vi "Construct_Optimal_Subtrack_(101-111)-1.vi"(6 "[IN] Indexes for Jumps":i32[](array[numeric]), 8 "error IN":errorcluster, 9 "[IN] Index of recon\nstructed tracks":i32, 10 "[IN] Clusters for Re\nconstructed Tracks":T1, 11 "[IN] Still connected\ntracks in group":T2) -> (0 "error OUT":errorcluster, 2 "[OUT] Clusters for Re\nconstructed Tracks":T1)   [LabVIEW 2013]
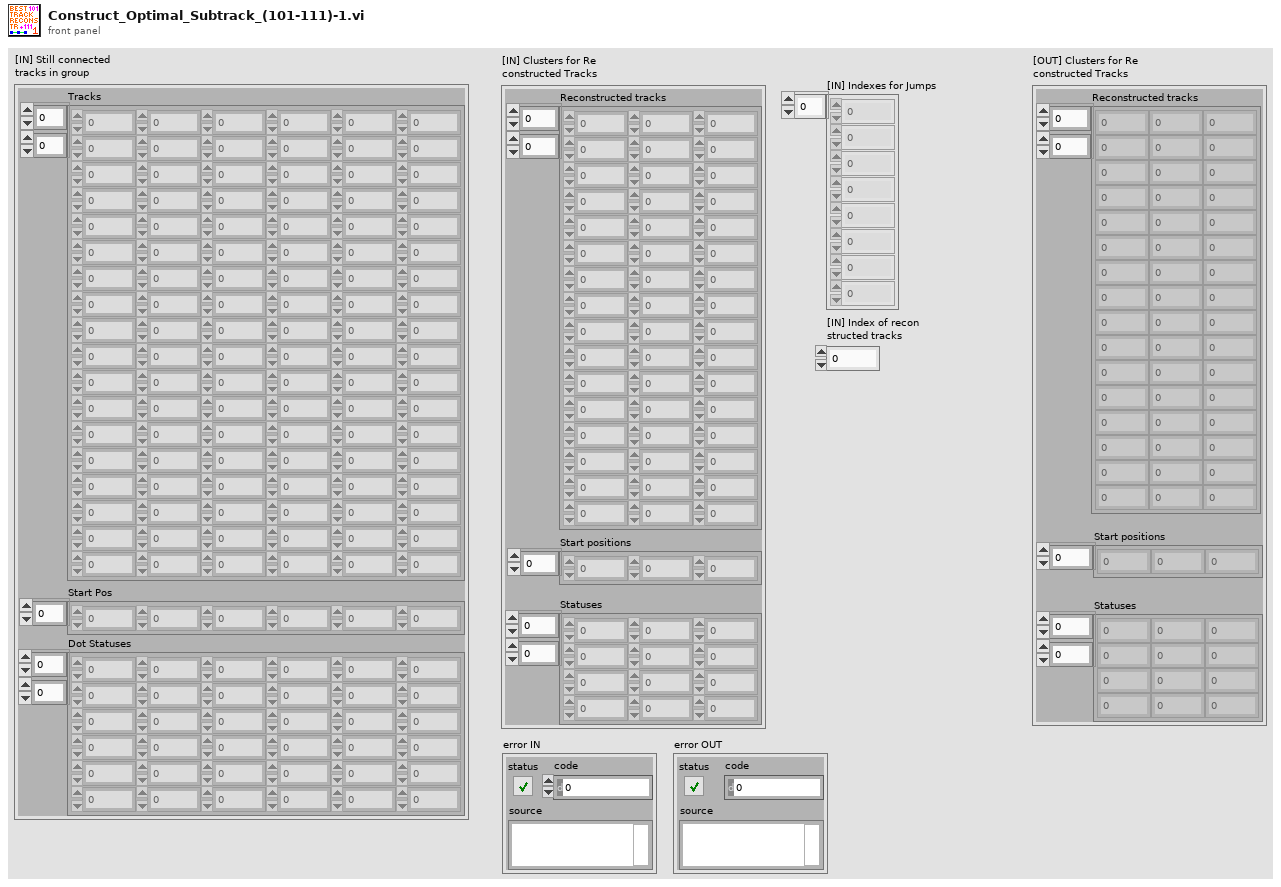
[diagram p1: front panel]
types:
  T1 = cluster{"Reconstructed tracks":dbl[][], "Start positions":i32[], "Statuses":i16[][]}
  T2 = cluster{"Tracks":dbl[][], "Start Pos":i32[], "Dot Statuses":i16[][]}
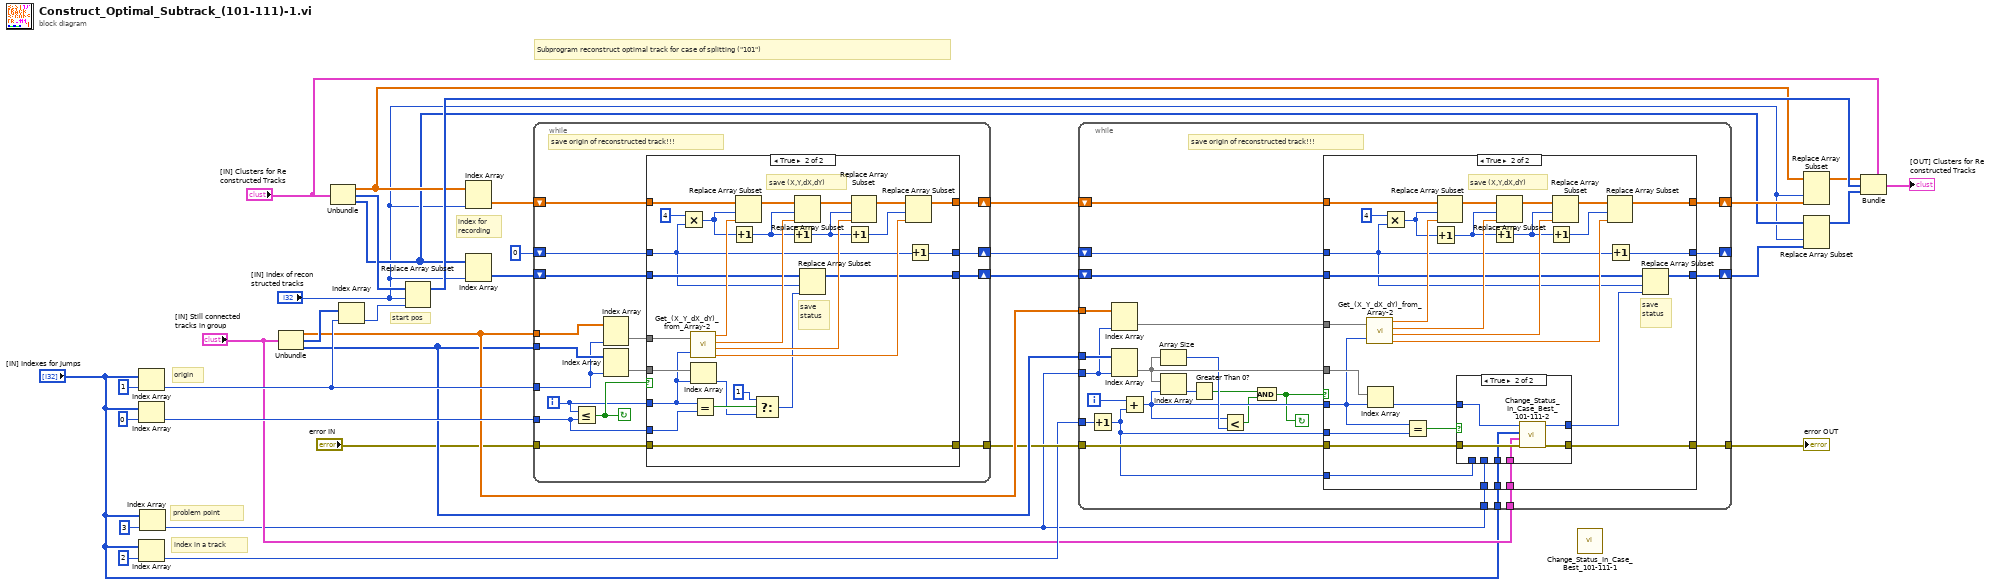
[diagram p0: block diagram]
diagram:
  # "index in a track"
  # "problem point"
  # "origin"
  # "Subprogram reconstruct optimal track for case of splitting (\"101\")"
  # "index for\nrecording"
  # "start pos"
  n1 = Index Array(array="[IN] Indexes for Jumps", index=1) -> (element=w27:i32)
  n2 = Index Array(array="[IN] Indexes for Jumps", index=0) -> (element=w30:i32)
  n3 = Index Array(array="[IN] Indexes for Jumps", index=2) -> (element=w7:i32)
  n4 = Index Array(array="[IN] Indexes for Jumps", index=3) -> (element=w3:i32)
  n5 = Unbundle("[IN] Still connected\ntracks in group") -> ("Tracks"=w19:dbl[][], "Start Pos"=w28:i32[], "Dot Statuses"=w18:i16[][])
  n6 = Unbundle("[IN] Clusters for Re\nconstructed Tracks") -> ("Reconstructed tracks"=w15:dbl[][], "Start positions"=w29:i32[], "Statuses"=w12:i16[][])
  n7 = Index Array(array=w28, index=w27) -> (element=w26:i32)
  n8 = Replace Array Subset(array=w29, new element=w26, index="[IN] Index of recon\nstructed tracks") -> (w16:i32[])
  n9 = Index Array(array=w15, index (col)="[IN] Index of recon\nstructed tracks") -> (element=w25:dbl[])  [unwired: 1 in]
  n10 = Index Array(array=w12, index (col)="[IN] Index of recon\nstructed tracks") -> (element=w24:i16[])  [unwired: 1 in]
  n11 = while {
    tunnel: w30 -> [w35]
    tunnel: w19 -> [w50]
    tunnel: w18 -> [w49]
    tunnel: w27 -> [w48]
    shift-right: [w40] -> w22
    shift-left: w25 -> [w46]
    shift-right: [w38] -> w20
    shift-left: w24 -> [w42]
    shift-right: [w39] -> w21
    shift-left: 0 -> [w41]
    tunnel: "error IN" -> [w37]
    tunnel: [w36] -> w8
    i -> [w43]
    stop <- w47 continue-if-true
    # "save origin of reconstructed track!!!"
    n12 = Less Or Equal?(x=w43, y=w35) -> (x <= y?=w47:bool)
    n13 = Index Array(array=w50, index (col)=w48) -> (element=w45:dbl[])  [unwired: 1 in]
    n14 = Index Array(array=w49, index (col)=w48) -> (element=w44:i16[])  [unwired: 1 in]
    n15 = case shown="True" w47 {
      tunnel: w46 -> [w54 w79]
      tunnel: w45 -> [_ w81]
      tunnel: w44 -> [_ w80]
      tunnel: w43 -> [_ w58]
      tunnel: w42 -> [w52 w66]
      tunnel: [w52 w65] -> w38
      tunnel: [w54 w64] -> w40
      tunnel: w41 -> [w53 w63]
      tunnel: [w53 w62] -> w39
      tunnel: w37 -> [w51 w61]
      tunnel: [w51 w61] -> w36
      tunnel: w35 -> [_ w57]
      frame False {
      }
      frame True {
        # "save (X,Y,dX,dY)"
        # "save\nstatus"
        n16 = Multiply(x=4, y=w63) -> (x*y=w75:i32)
        n17 = call "Get_(X_Y_dX_dY)_from_Array-2.vi"("(X,Y,dX,dY)"=w81, "Index of Displacement"=w58) -> ("X"=w77:dbl, "Y"=w74:dbl, "dX"=w71:dbl, "dY"=w67:dbl)
        n18 = Index Array(array=w80, index=w58) -> (element=w55:i16)
        n19 = Equal?(x=w58, y=w57) -> (x = y?=w59:bool)
        n20 = Increment(x=w75) -> (x+1=w72:i32)
        n21 = Replace Array Subset(array=w79, new element=w77, index=w75) -> (w76:dbl[])
        n22 = Select(t=i16 1, s=w59, f=w55) -> (s? t:f=w56:i16)
        n23 = Increment(x=w72) -> (x+1=w70:i32)
        n24 = Replace Array Subset(array=w76, new element=w74, index=w72) -> (w73:dbl[])
        n25 = Replace Array Subset(array=w66, new element=w56, index=w63) -> (w65:i16[])
        n26 = Increment(x=w70) -> (x+1=w69:i32)
        n27 = Replace Array Subset(array=w73, new element=w71, index=w70) -> (w68:dbl[])
        n28 = Replace Array Subset(array=w68, new element=w67, index=w69) -> (w64:dbl[])
        n29 = Increment(x=w63) -> (x+1=w62:i32)
      }
    }
  }
  n30 = while {
    tunnel: w19 -> [w106]
    tunnel: w18 -> [w105]
    tunnel: w3 -> [w84]
    shift-right: [w100] -> w14
    shift-left: w22 -> [w104]
    shift-right: [w98] -> w11
    shift-left: w20 -> [w102]
    shift-right: [w99] -> _
    shift-left: w21 -> [w101]
    tunnel: w7 -> [w87]
    tunnel: w8 -> [w89]
    tunnel: [w88] -> w2
    tunnel: "[IN] Still connected\ntracks in group" -> [w86]
    tunnel: w3 -> [w83]
    tunnel: "[IN] Indexes for Jumps" -> [w82]
    i -> [w97]
    stop <- w90 continue-if-true
    # "save origin of reconstructed track!!!"
    n31 = Increment(x=w87) -> (x+1=w85:i32)
    n32 = Index Array(array=w106, index (col)=w84) -> (element=w103:dbl[])  [unwired: 1 in]
    n33 = Index Array(array=w105, index (col)=w84) -> (element=w96:i16[])  [unwired: 1 in]
    n34 = Add(x=w97, y=w85) -> (x+y=w93:i32)
    n35 = Array Size(array=w96) -> (size(s)=w94:i32)
    n36 = Index Array(array=w96, index=w93) -> (element=w95:i16)
    n37 = Greater Than 0?(x=w95) -> (x > 0?=w92:bool)
    n38 = Less?(x=w93, y=w94) -> (x < y?=w91:bool)
    n39 = And(x=w92, y=w91) -> (x .and. y?=w90:bool)
    n40 = case shown="True" w90 {
      tunnel: w104 -> [w110 w140]
      tunnel: w103 -> [_ w141]
      tunnel: w96 -> [_ w122]
      tunnel: w93 -> [_ w121]
      tunnel: w102 -> [w108 w127]
      tunnel: [w108 w126] -> w98
      tunnel: [w110 w125] -> w100
      tunnel: w101 -> [w109 w124]
      tunnel: [w109 w123] -> w99
      tunnel: w89 -> [w107 w118]
      tunnel: [w107 w116] -> w88
      tunnel: w85 -> [_ w120]
      tunnel: w86 -> [_ w114]
      tunnel: w85 -> [_ w113]
      tunnel: w83 -> [_ w112]
      tunnel: w82 -> [_ w111]
      frame False {
      }
      frame True {
        # "save (X,Y,dX,dY)"
        # "save\nstatus"
        n41 = call "Get_(X_Y_dX_dY)_from_Array-2.vi"("(X,Y,dX,dY)"=w141, "Index of Displacement"=w121) -> ("X"=w138:dbl, "Y"=w135:dbl, "dX"=w132:dbl, "dY"=w128:dbl)
        n42 = Index Array(array=w122, index=w121) -> (element=w117:i16)
        n43 = Multiply(x=4, y=w124) -> (x*y=w136:i32)
        n44 = Equal?(x=w121, y=w120) -> (x = y?=w119:bool)
        n45 = Increment(x=w136) -> (x+1=w133:i32)
        n46 = Replace Array Subset(array=w140, new element=w138, index=w136) -> (w137:dbl[])
        n47 = case shown="True" w119 {
          tunnel: w118 -> [w143 w149]
          tunnel: w117 -> [w142 w147]
          tunnel: [w142 w148] -> w115
          tunnel: [w143 w145] -> w116
          tunnel: w114 -> [_ w146]
          tunnel: w113 -> [_ _]
          tunnel: w112 -> [_ _]
          tunnel: w111 -> [_ w144]
          frame False {
          }
          frame True {
            n48 = call "Change_Status_In_Case_Best_101-111-2.vi"("error IN"=w149, "[IN] Track group"=w146, "[IN] Indexes for Jumps"=w144, "[IN] Current Status"=w147) -> ("error OUT"=w145:errorcluster, "[OUT] Status of point after 101"=w148:i16)  [unwired: 3 in]
          }
        }
        n49 = Increment(x=w133) -> (x+1=w131:i32)
        n50 = Replace Array Subset(array=w137, new element=w135, index=w133) -> (w134:dbl[])
        n51 = Increment(x=w131) -> (x+1=w130:i32)
        n52 = Replace Array Subset(array=w134, new element=w132, index=w131) -> (w129:dbl[])
        n53 = Replace Array Subset(array=w129, new element=w128, index=w130) -> (w125:dbl[])
        n54 = Increment(x=w124) -> (x+1=w123:i32)
        n55 = Replace Array Subset(array=w127, new element=w115, index=w124) -> (w126:i16[])
      }
    }
  }
  "error OUT" <- w2
  n56 = call "Change_Status_In_Case_Best_101-111-1.vi"() -> ()  [unwired: 7 in, 2 out]
  n57 = Replace Array Subset(array=w15, new element=w14, index (col)="[IN] Index of recon\nstructed tracks") -> (w13:dbl[][])  [unwired: 1 in]
  n58 = Replace Array Subset(array=w12, new element=w11, index (col)="[IN] Index of recon\nstructed tracks") -> (w5:i16[][])  [unwired: 1 in]
  n59 = Bundle(cluster="[IN] Clusters for Re\nconstructed Tracks", "Reconstructed tracks"=w13, "Start positions"=w16, "Statuses"=w5) -> (→"[OUT] Clusters for Re\nconstructed Tracks":T1)
